vi "calibrating_dialog_popup.vi"(8 "error in (no error)":errorcluster) -> (0 "error out":errorcluster)   [LabVIEW 2016]
panel:
  out "Status":string="Shutting down...Sweeping field to zero..."
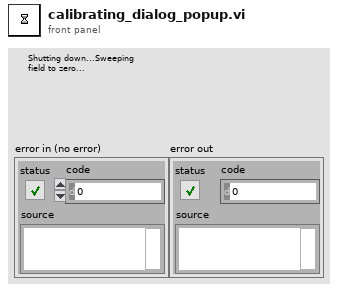
[diagram p1: front panel]
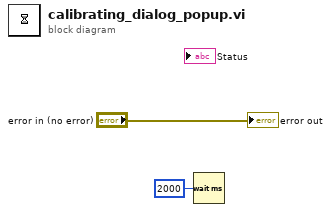
[diagram p0: block diagram]
diagram:
  n1 = Wait (ms)(milliseconds to wait=u32 2000) -> ()  [unwired: 1 out]
  "error out" <- "error in (no error)"
